vi "HXG2_Analog-IN_Final.vi"(8 "error in (no error)":errorcluster, 10 "ANALOG.Liq Mdot":dbl, 11 "MAX":T2) -> (0 "error out":errorcluster, 3 "ANALOG OUT":T1)   [LabVIEW 2012]
uses:
  Controls/HXG2_MaxConstants.ctl
  Controls/HXG2_AnalogIn.ctl
  <vilib>/DAQmx/read.llb/DAQmx Read (Analog 2D DBL NChan NSamp).vi
  <resource>/objmgr/daqmx.rc
panel:
  out "Input.OnbrdBufSize 2":u32
  out "Input.OnbrdBufSize":u32
  out "size(s)":i32[](array[numeric])
  out "Monitored Array":dbl[][](array[numeric])
  out "Taken TC":u32
  out "Taken Analog":u32
  out "AvailSamp Analog":u32
  out "AvailSamp TC":u32
  out "State Execution (ms)":u32 format="%.6p"
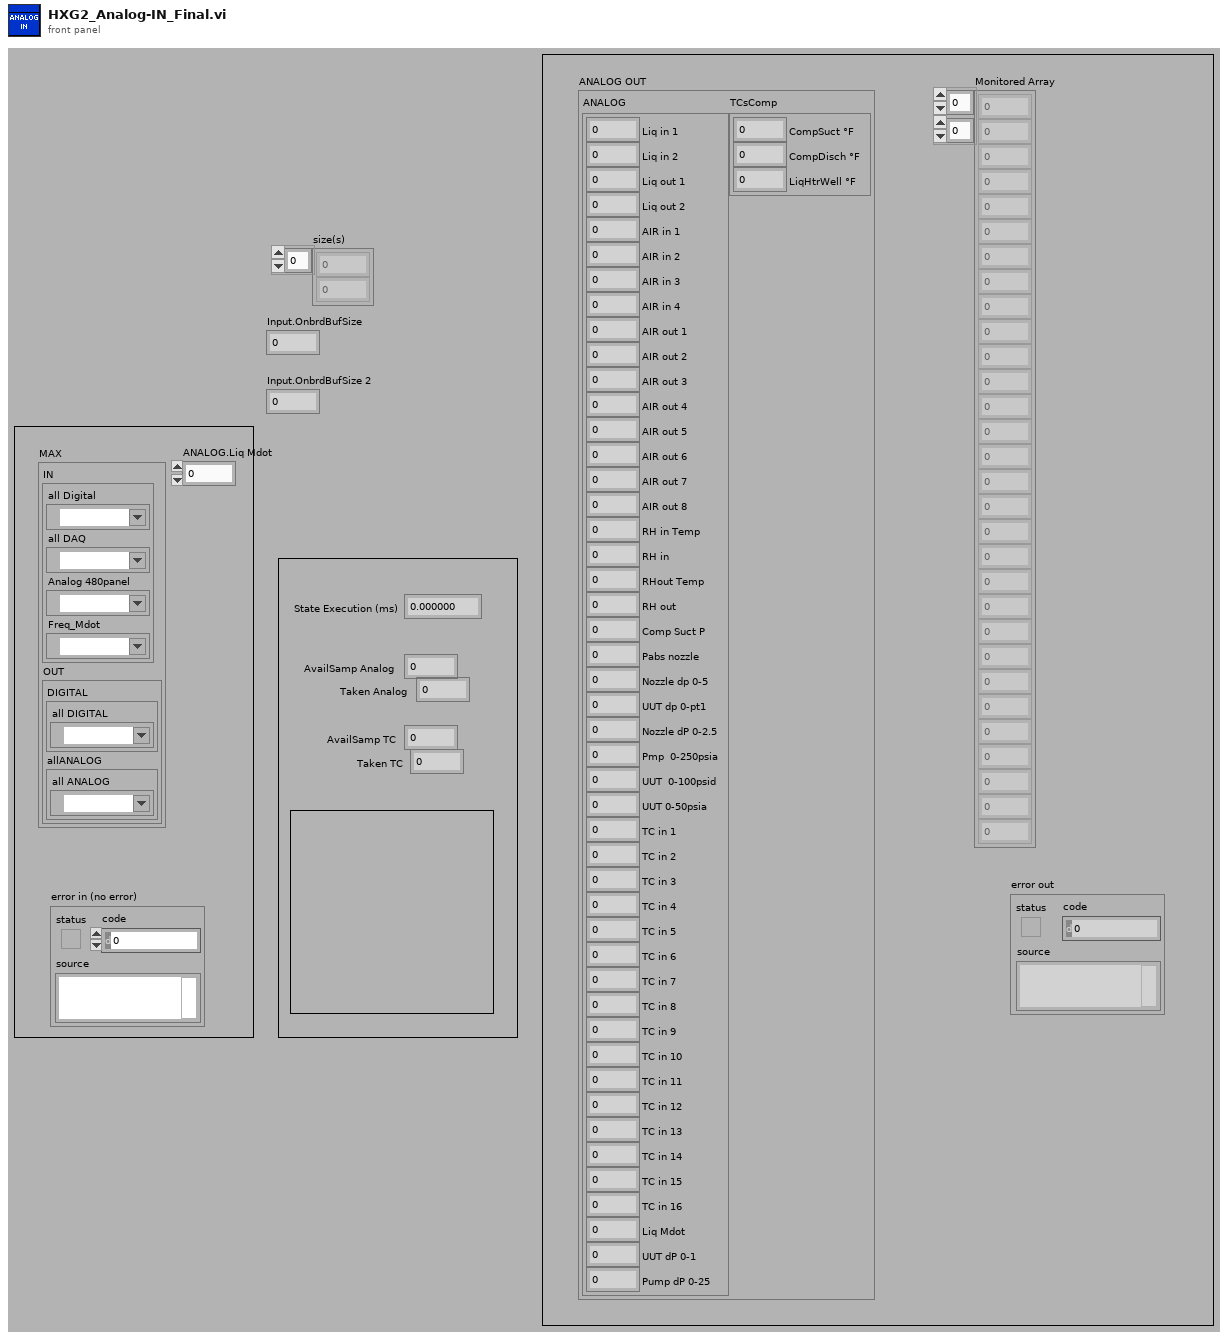
[diagram p1: front panel]
types:
  T1 = typedef "HXG2_AnalogIn.ctl" = cluster{"ANALOG":cluster{"Liq in 1":dbl, "Liq in 2":dbl, "Liq out 1":dbl, "Liq out 2":dbl, "AIR in 1":dbl, "AIR in 2":dbl, "AIR in 3":dbl, "AIR in 4":dbl, "AIR out 1":dbl, "AIR out 2":dbl, "AIR out 3":dbl, "AIR out 4":dbl, "AIR out 5":dbl, "AIR out 6":dbl, "AIR out 7":dbl, "AIR out 8":dbl, "RH in Temp":dbl, "RH in":dbl, "RHout Temp":dbl, "RH out":dbl, "Comp Suct P":dbl, "Pabs nozzle":dbl, "Nozzle dp 0-5":dbl, "UUT dp 0-pt1":dbl, "Nozzle dP 0-2.5":dbl, "Pmp  0-250psia":dbl, "UUT  0-100psid":dbl, "UUT 0-50psia":dbl, "TC in 1":dbl, "TC in 2":dbl, "TC in 3":dbl, "TC in 4":dbl, "TC in 5":dbl, "TC in 6":dbl, "TC in 7":dbl, "TC in 8":dbl, "TC in 9":dbl, "TC in 10":dbl, "TC in 11":dbl, "TC in 12":dbl, "TC in 13":dbl, "TC in 14":dbl, "TC in 15":dbl, "TC in 16":dbl, "Liq Mdot":dbl, "UUT dP 0-1":dbl, "Pump dP 0-25":dbl}, "TCsComp":cluster{"CompSuct °F  ":dbl, "CompDisch °F":dbl, "LiqHtrWell °F":dbl}}
  T2 = typedef "HXG2_MaxConstants.ctl" = cluster{"IN":cluster{"all Digital":refnum<k21>, "all DAQ":refnum<k21>, "Analog 480panel":refnum<k21>, "Freq_Mdot":refnum<k21>}, "OUT":cluster{"DIGITAL":cluster{"all DIGITAL":refnum<k21>}, "allANALOG":cluster{"all ANALOG":refnum<k21>}}}
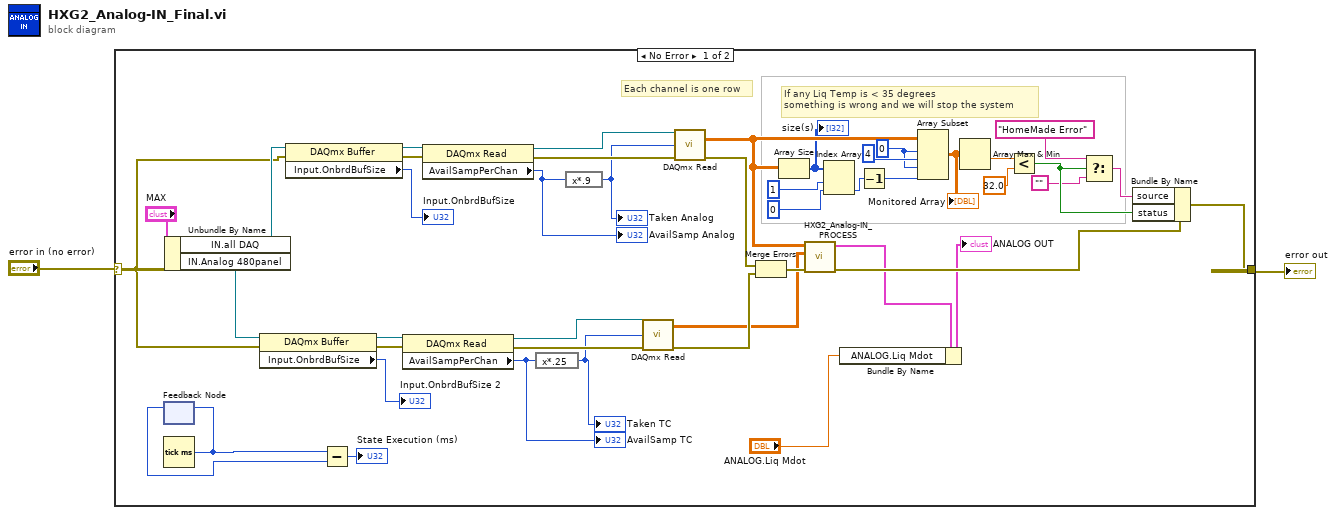
[diagram p0: block diagram]
diagram:
  n1 = case shown="No Error" "error in (no error)" {
    selector: "error in (no error)" -> [w9 w48]
    tunnel: [w23 w48] -> w1
    frame No Error {
      w20 = 0 ("index")
      # "Each channel is one row"
      # "If any Liq Temp is < 35 degrees\nsomething is wrong and we will stop the system"
      n2 = feedback #1() -> (w46:u32)  [unwired: 1 in]
      n3 = Tick Count (ms)() -> (millisecond timer value=w45:u32)
      n4 = feedback-in #1(w45) -> ()
      n5 = Unbundle By Name("MAX") -> ("IN.all DAQ"=w13:refnum<k21>, "IN.Analog 480panel"=w10:refnum<k21>)
      n6 = property class="DAQmx Buffer"(reference=w10, error in=w9) -> (reference out=w7:refnum<k21>, error out=w11:errorcluster, "Input.OnbrdBufSize"=→"Input.OnbrdBufSize 2":u32)
      n7 = property class="DAQmx Buffer"(reference=w13, error in=w9) -> (reference out=w14:refnum<k21>, error out=w3:errorcluster, "Input.OnbrdBufSize"=→"Input.OnbrdBufSize":u32)
      n8 = Subtract(x=w45, y=w46) -> (x-y=→"State Execution (ms)":u32)
      n9 = property class="DAQmx Read"(reference=w7, error in=w11) -> (reference out=w44:refnum<k21>, error out=w37:errorcluster, "AvailSampPerChan"=w36:u32)
      "AvailSamp TC" <- w36
      n10 = property class="DAQmx Read"(reference=w14, error in=w3) -> (reference out=w41:refnum<k21>, error out=w40:errorcluster, "AvailSampPerChan"=w35:u32)
      "AvailSamp Analog" <- w35
      n11 = expression code="x*.25"(w36) -> (w32:u32)
      "Taken TC" <- w32
      n12 = expression code="x*.9"(w35) -> (w38:u32)
      "Taken Analog" <- w38
      n13 = call-poly <vilib>:"DAQmx Read.vi"("task/channels in"=w44, "number of samples per channel"=w32, "error in"=w37) -> ("data"=w34:dbl[][], "error out"=w42:errorcluster)  [unwired: 10 in, 1 out]
      n14 = call-poly <vilib>:"DAQmx Read.vi"("task/channels in"=w41, "number of samples per channel"=w38, "error in"=w40) -> ("data"=w31:dbl[][], "error out"=w43:errorcluster)  [unwired: 10 in, 1 out]
      n15 = Merge Errors(w43, w42) -> (w39:errorcluster)
      n16 = Array Size(array=w31) -> (size(s)=w30:i32[])
      "size(s)" <- w30
      n17 = call "HXG2_Analog-IN_PROCESS.vi"("error in (no error)"=w39, "Analog TC"=w34, "Analog In"=w31) -> ("error out"=w24:errorcluster, "ANALOG OUT"=w6:T1)  [unwired: 7 in]
      n18 = Index Array(array=w30, index #1=1 ("index"), index #2=0 ("index")) -> (element #2=w22:i32)  [unwired: 1 out]
      n19 = Bundle By Name(cluster=w6, "ANALOG.Liq Mdot"="ANALOG.Liq Mdot") -> (→"ANALOG OUT":T1)
      n20 = Decrement(x=w22) -> (x-1=w19:i32)
      n21 = Array Subset(array=w31, index (row)=w20, length (row)=4 ("index"), index (col)=w20, length (col)=w19) -> (w27:dbl[][])
      "Monitored Array" <- w27
      n22 = Array Max & Min(array=w27) -> (min value=w26:dbl)  [unwired: 3 out]
      n23 = Less?(x=w26, y=32.0) -> (x < y?=w18:bool)
      n24 = Select(t="HomeMade Error", s=w18, f="") -> (s? t:f=w17:string)
      n25 = Bundle By Name(cluster=w24, "source"=w17, "status"=w18) -> (w23:errorcluster)
    }
    frame Error {
    }
  }
  "error out" <- w1
